vi "Normal Drive (Autonomous).vi"(1 "Execute":bool=TRUE, 2 "Distance (Feet)":dbl=10.0, 3 "Percent Speed":dbl=0.8) -> (4 "Done Executing":bool, 6 "x >= y?":bool, 7 "abs(x)":dbl, 8 "abs(x) 2":dbl)   [LabVIEW 2011]
uses:
  Globals/Encoders Global.vi
  Globals/Autonomous Joystick Emulation.vi
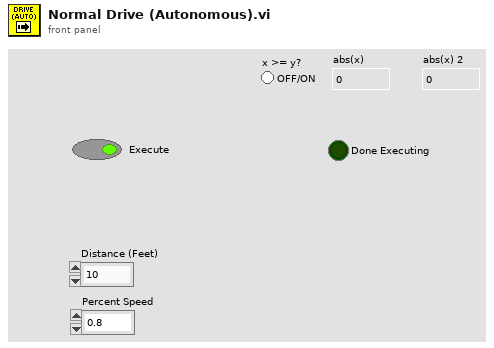
[diagram p1: front panel]
types:
  T1 = typedef "WPI_EncoderDevRef.ctl" = cluster{"DevStatus":errorcluster, "EncoderIndex":T2, "CounterIndex":T3, "DistancePerCount":dbl, "Decoding Type":T4}
  T2 = typedef "FPGA_EncoderIdx.ctl" = enum8{"Enc 0", "Enc 1", "Enc 2", "Enc 3", "Invalid"}
  T3 = typedef "FPGA_CounterCtrSystemIndex.ctl" = enum8{"Ctr 0", "Ctr 1", "Ctr 2", "Ctr 3", "Ctr 4", "Ctr 5", "Ctr 6", "Ctr 7", "Invalid"}
  T4 = typedef "WPI_EncoderType.ctl" = enum16{"1x", "2x", "4x"}
  T5 = cluster{"Front Left":T1, "Front Right":T1, "Rear Left":T1, "Rear Right":T1, "Shooter":T1}
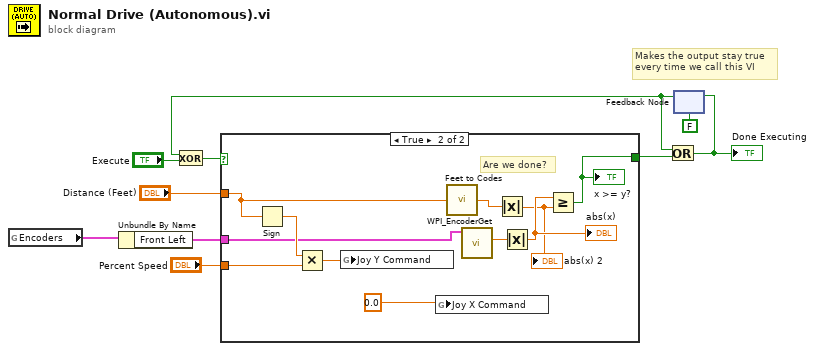
[diagram p0: block diagram]
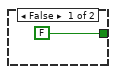
[diagram p2: hidden frame]
diagram:
  # "Makes the output stay true\nevery time we call this VI"
  n1 = global read "Encoders Global.vi" "Encoders"() -> (w4:T5)
  n2 = Unbundle By Name(w4) -> ("Front Left"=w3:T1)
  n3 = feedback #1(FALSE) -> (w1:bool)
  n4 = Exclusive Or(1:"Execute", 2:w1) -> (0:w10:bool)
  n5 = case shown="True" w10 {
    tunnel: [FALSE w22] -> w8
    tunnel: "Percent Speed" -> [_ w19]
    tunnel: "Distance (Feet)" -> [_ w18]
    tunnel: w3 -> [_ w12]
    frame False {
    }
    frame True {
      # "Are we done?"
      n6 = Sign(1:w18) -> (0:w17:dbl)
      n7 = Multiply(x=w17, y=w19) -> (x*y=w14:dbl)
      n8 = global write "Autonomous Joystick Emulation.vi" "Joy Y Command"(w14) -> ()
      n9 = global write "Autonomous Joystick Emulation.vi" "Joy X Command"(0.0 ("Joy X Command")) -> ()
      n10 = call "Feet to Codes.vi"("Feet"=w18) -> ("Codes"=w21:dbl)
      n11 = call <vilib>:"WPI_EncoderGet.vi"("EncoderDevRef"=w12) -> ("Distance"=w20:dbl)  [unwired: 5 in, 5 out]
      n12 = Absolute Value(x=w21) -> (abs(x)=w15:dbl)
      "abs(x) 2" <- w15
      n13 = Absolute Value(x=w20) -> (abs(x)=w16:dbl)
      "abs(x)" <- w16
      n14 = Greater Or Equal?(x=w16, y=w15) -> (x >= y?=w22:bool)
      "x >= y?" <- w22
    }
  }
  n15 = Or(x=w1, y=w8) -> (x .or. y?=w2:bool)
  "Done Executing" <- w2
  n16 = feedback-in #1(w2) -> ()
